vi "RPI_SenseHat_Server.vi"() -> ()   [LabVIEW 2020]
uses:
  Classes/RaspberryPi Actor/RaspberryPi Actor.lvclass
  C:/Program Files (x86)/National Instruments/LabVIEW 2020/vi.lib/ActorFramework/Actor/Actor.lvclass
  <vilib>/ActorFramework/Message Enqueuer/Message Enqueuer.lvclass/Message Enqueuer.ctl
  Classes/RaspberryPi Actor Messages/Set LED Display Msg/Set LED Display Msg.lvclass/Set LED Display Msg.ctl
  <vilib>/ActorFramework/Message Enqueuer/Enqueue.vi
  Classes/RaspberryPi Actor Messages/New LED Display Msg/New LED Display Msg.lvclass
  C:/Program Files (x86)/National Instruments/LabVIEW 2020/vi.lib/ActorFramework/Message/Message.lvclass
  Classes/RaspberryPi Actor Messages/Clear LED Display Msg/Clear LED Display Msg.lvclass
  Classes/RaspberryPi Actor Messages/Stop LED Display Msg/Stop LED Display Msg.lvclass
  Classes/RaspberryPi Actor Messages/Set LED Display Msg/Set LED Display Msg.lvclass
  <vilib>/ActorFramework/Stop Msg/Stop Msg.lvclass
  <vilib>/ActorFramework/Message Priority Queue/Priority Enqueue.vi
  <vilib>/ActorFramework/Actor/Actor.lvclass
panel:
  in  "setLEDDisplay":bool
  in  "LED Display":u32[][](array[colorbox])=[[0, 0, 0, 0, 0, 0, 0, 0], [0, 0, 0, 0, 0, 0, 0, 0], [0, 0, 0, 0, 0, 0, 0, 0], [0, 0, 0, 0, 0, 0, 0, 0], [0, 0, 0, 0, 0, 0, 0, 0], [0, 0, 0, 0, 0, 0, 0, 0], [0, 0, 0, 0, 0, 0, 0, 0], [0, 0, 0, 0, 0, 0, 0, 0], [0, 0, 0, 0, 0, 0, 0, 0]]
  in  "stopLEDDisplay":bool
  in  "clearLEDDisplay":bool
  in  "newLEDDisplay":bool
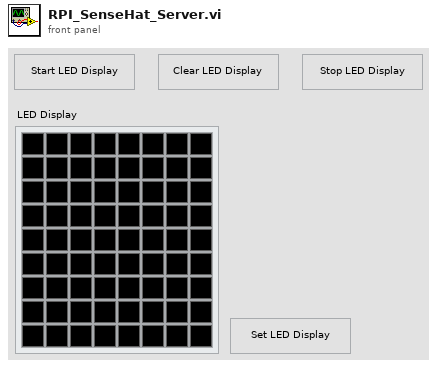
[diagram p1: front panel]
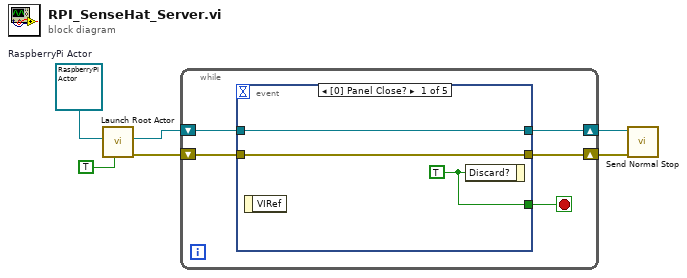
[diagram p0: block diagram]
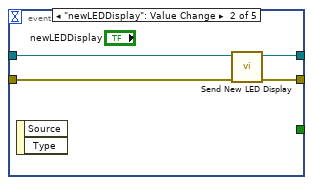
[diagram p2: hidden frame]
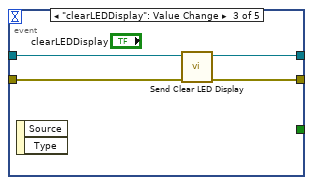
[diagram p3: hidden frame]
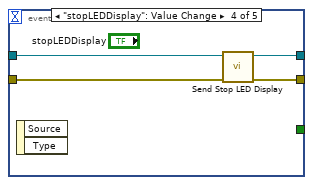
[diagram p4: hidden frame]
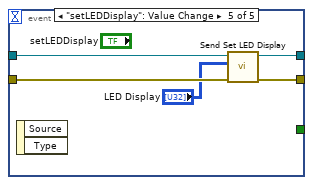
[diagram p5: hidden frame]
diagram:
  w6 = refnum<class "RaspberryPi Actor.lvclass"> refnum  # RaspberryPi Actor
  n1 = call <vilib>:"Launch Root Actor.vi"("Open Actor Core front panel? (F)"=TRUE, "Actor"=w6) -> ("error out"=w4:errorcluster, "Actor's Enqueuer"=w5:refnum<class "Message Enqueuer.lvclass">)  [unwired: 8 in]
  n2 = while {
    shift-right: [w7] -> w2
    shift-left: w4 -> [w8]
    shift-right: [w10] -> w3
    shift-left: w5 -> [w11]
    stop <- w9 stop-if-true
    n3 = event shown="[0] Panel Close?" {
      selector: _ -> [_ _ _ _ _]
      dyn-events: _ -> [_ _ _ _ _]
      timeout: _ -> [_ _ _ _ _]
      tunnel: w11 -> [w14 w18 w22 w26 w31]
      tunnel: [w14 w17 w21 w25 w29] -> w10
      tunnel: [w13 _ _ _ _] -> w9
      tunnel: w8 -> [w12 w15 w19 w24 w30]
      tunnel: [w12 w16 w20 w23 w28] -> w7
      event Panel Close? {
        w13 = TRUE ("Discard?")
        n4 = event-data() -> ()  [unwired: 1 in, 1 out]
        n5 = event-data("Discard?"=w13) -> ()  [unwired: 1 in, 1 out]
      }
      event "newLEDDisplay": Value Change {
        n6 = event-data() -> ()  [unwired: 1 in, 2 out]
        n7 = call "Send New LED Display.vi"("error in (no error)"=w15, "Message Enqueuer"=w18) -> ("error out"=w16:errorcluster, "Message Enqueuer out"=w17:refnum<class "Message Enqueuer.lvclass">)  [unwired: 8 in]
      }
      event "clearLEDDisplay": Value Change {
        n8 = event-data() -> ()  [unwired: 1 in, 2 out]
        n9 = call "Send Clear LED Display.vi"("error in (no error)"=w19, "Message Enqueuer"=w22) -> ("error out"=w20:errorcluster, "Message Enqueuer out"=w21:refnum<class "Message Enqueuer.lvclass">)  [unwired: 8 in]
      }
      event "stopLEDDisplay": Value Change {
        n10 = event-data() -> ()  [unwired: 1 in, 2 out]
        n11 = call "Send Stop LED Display.vi"("error in (no error)"=w24, "Message Enqueuer"=w26) -> ("error out"=w23:errorcluster, "Message Enqueuer out"=w25:refnum<class "Message Enqueuer.lvclass">)  [unwired: 8 in]
      }
      event "setLEDDisplay": Value Change {
        n12 = event-data() -> ()  [unwired: 1 in, 2 out]
        n13 = call "Send Set LED Display.vi"("error in (no error)"=w30, "LED Matrix"="LED Display", "Message Enqueuer"=w31) -> ("error out"=w28:errorcluster, "Message Enqueuer out"=w29:refnum<class "Message Enqueuer.lvclass">)  [unwired: 7 in]
      }
    }
  }
  n14 = call <vilib>:"Send Normal Stop.vi"("error in (no error)"=w2, "Message Enqueuer"=w3) -> ()  [unwired: 9 in, 1 out]
